vi "Convert SGL to FXP.vi"(7 "Input":sgl) -> (6 "U32":u32, 8 "FXP Output":fxp<+,32,32>, 10 "I32":i32)   [LabVIEW 2012]
uses:
  <vilib>/rvi/FXPMathLib/FxpInterpret/XNode/nifxpmath_Interpret.xnode
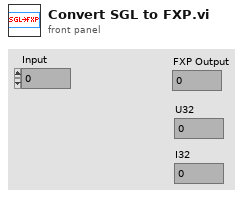
[diagram p1: front panel]
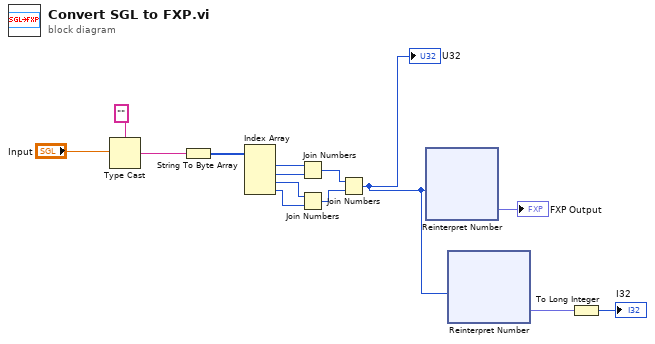
[diagram p0: block diagram]
diagram:
  n1 = Type Cast(type="", x="Input") -> (*(type *) &x=w13:string)
  n2 = String To Byte Array(string=w13) -> (unsigned byte array=w12:u8[])
  n3 = Index Array(array=w12) -> (element #1=w10:u8, element #2=w11:u8, element #3=w9:u8, element #4=w8:u8)  [unwired: 4 in]
  n4 = Join Numbers(hi=w10, lo=w11) -> ((hi.lo)=w6:u16)
  n5 = Join Numbers(hi=w9, lo=w8) -> ((hi.lo)=w7:u16)
  n6 = Join Numbers(hi=w6, lo=w7) -> ((hi.lo)=w3:u32)
  "U32" <- w3
  n7 = xnode "Reinterpret Number"("x"=w3) -> ("y"=→"FXP Output":fxp<+,32,32>)
  n8 = xnode "Reinterpret Number"("x"=w3) -> ("y"=w2:fxp<+/-,32,32>)
  n9 = To Long Integer(number=w2) -> (32bit integer=→"I32":i32)
